vi "NanonisFrame-Demod.vi"(0 "x":dbl, 1 "z":dbl) -> (8 "X Out":dbl, 10 "Z Out":dbl, 12 "Speed":dbl, 14 "FO X":dbl, 15 "FO Z":dbl, 16 "FW":dbl, 17 "FH":dbl, 19 "CVAL (nA)":dbl)   [LabVIEW 2017]
uses:
  <userlib>/Nanonis Prog Interface V5/Nanonis Prog Interface.lvlib
panel:
  out "Signal value":sgl format="%#_6p"
  out "Signals Names":string[](array[string])
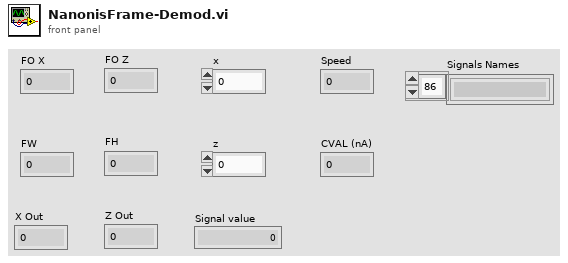
[diagram p1: front panel]
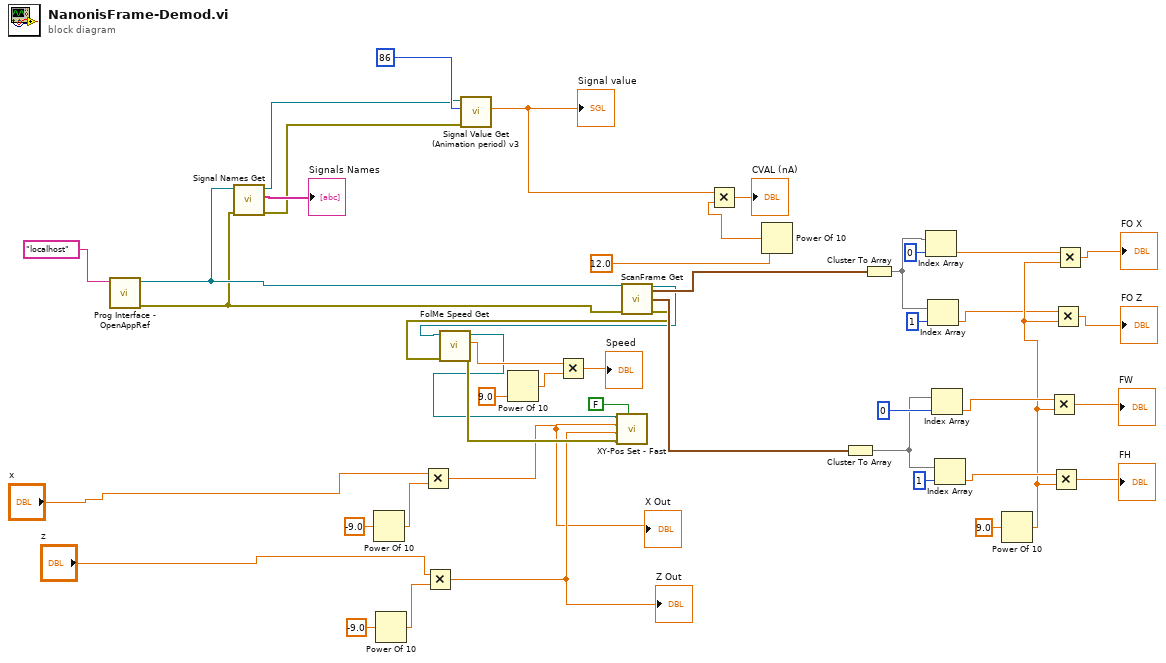
[diagram p0: block diagram]
diagram:
  n1 = call <userlib>:"Prog Interface - OpenAppRef.vi"("Machine name (local machine IP)"="localhost") -> ("Error out"=w5:errorcluster, "Application reference"=w6:refnum<vi>)  [unwired: 5 in]
  n2 = call <userlib>:"Signal Names Get.vi"("error in (no error)"=w5, "Application ref in"=w6) -> ("error out"=w3:errorcluster, "Signals Names"=→"Signals Names":string[], "Application ref out"=w2:refnum<vi>)  [unwired: 5 in]
  n3 = Power Of 10(x=-9.0) -> (10^x=w26:dbl)
  n4 = Power Of 10(x=-9.0) -> (10^x=w24:dbl)
  n5 = Multiply(x="x", y=w26) -> (x*y=w10:dbl)
  "X Out" <- w10
  n6 = Multiply(x="z", y=w24) -> (x*y=w11:dbl)
  "Z Out" <- w11
  n7 = call <userlib>:"Signal Value Get (Animation period) v3.vi"("error in (no error)"=w3, "Signal index (0-127)"=i8 86, "Application ref in"=w2) -> ("Signal value"=w1:sgl)  [unwired: 5 in, 2 out]
  "Signal value" <- w1
  n8 = Power Of 10(x=9.0) -> (10^x=w29:dbl)
  n9 = call <userlib>:"ScanFrame Get.vi"("Application ref in"=w6, "error in (no error)"=w5) -> ("Application ref out"=w31:refnum<vi>, "Center coordinates (m)"=w45:cluster{"Xc":sgl, "Yc":sgl}, "Size (m)"=w41:cluster{"Width":sgl, "Height":sgl}, "error out"=w22:errorcluster)  [unwired: 9 in, 1 out]
  n10 = call <userlib>:"FolMe Speed Get.vi"("error in (no error)"=w22, "Application ref in"=w31) -> ("error out"=w12:errorcluster, "Speed (m/s)"=w28:sgl, "Application ref out"=w9:refnum<vi>)  [unwired: 4 in, 1 out]
  n11 = Multiply(x=w28, y=w29) -> (x*y=→"Speed":dbl)
  n12 = call <userlib>:"XY-Pos Set - Fast.vi"("Wait end-of-motion (T=True)"=FALSE, "error in (no error)"=w12, "Y (m)"=w11, "X (m)"=w10, "Application ref in"=w9) -> ()  [unwired: 4 in, 2 out]
  n13 = Power Of 10(x=12.0) -> (10^x=w14:dbl)
  n14 = Multiply(x=w1, y=w14) -> (x*y=→"CVAL (nA)":dbl)
  n15 = Cluster To Array(cluster=w41) -> (array=w38:sgl[])
  n16 = Cluster To Array(cluster=w45) -> (array=w44:sgl[])
  n17 = Index Array(array=w44, index=0) -> (element=w19:sgl)
  n18 = Index Array(array=w44, index=1) -> (element=w18:sgl)
  n19 = Index Array(array=w38, index=0) -> (element=w37:sgl)
  n20 = Index Array(array=w38, index=1) -> (element=w36:sgl)
  n21 = Power Of 10(x=9.0) -> (10^x=w34:dbl)
  n22 = Multiply(x=w37, y=w34) -> (x*y=→"FW":dbl)
  n23 = Multiply(x=w36, y=w34) -> (x*y=→"FH":dbl)
  n24 = Multiply(x=w18, y=w34) -> (x*y=→"FO Z":dbl)
  n25 = Multiply(x=w19, y=w34) -> (x*y=→"FO X":dbl)
